vi "Set Sif Comment.vi"(11 "comment":string) -> (2 "function return":u32, 3 "comment out":string)   [LabVIEW 2018, in "Copy of Andor SDK.lvlib"]
doc: "EXPNETTYPE unsigned int WINAPI SetSifComment(char * comment);"
uses:
  Copy of Andor SDK.lvlib
  <userlib>/Andor SDK/ATMCD32D.dll
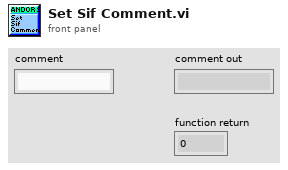
[diagram p1: front panel]
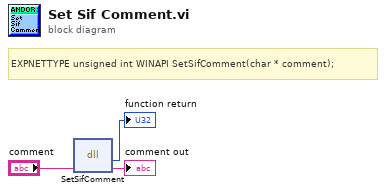
[diagram p0: block diagram]
diagram:
  # "EXPNETTYPE unsigned int WINAPI SetSifComment(char * comment);"
  n1 = dll-call lib="C:/Program Files (x86)/National Instruments/LabVIEW 2018/user.lib/Andor SDK/ATMCD32D.*" fn="SetSifComment"("comment"="comment") -> (→"function return":u32, "comment"=→"comment out":string)  [unwired: 3 in, 2 out]
